vi "Set Relay State.vi"(8 "error in (no error)":errorcluster, 9 "relay action (Close Relay)":T1=enum."Close Relay", 10 "SLSC Switch in":refnum<class "SLSC Switch.lvclass">, 11 "DevicePropertyRelay in":refnum<class "DevicePropertyRelay.lvclass">) -> (0 "error out":errorcluster, 2 "SLSC Switch out":refnum<class "SLSC Switch.lvclass">, 3 "DevicePropertyRelay out":refnum<class "DevicePropertyRelay.lvclass">)   [LabVIEW 2015, in "DevicePropertyRelay.lvclass"]
uses:
  DevicePropertyRelay.lvclass
  slscsl/RelayAction.ctl
  SLSC Switch/SLSC Switch.lvclass
  SLSC Switch/SLSC Switch.lvclass/SLSC Switch.ctl
  DevicePropertyRelay.lvclass/DevicePropertyRelay.ctl
  <vilib>/SLSC/Set Device Property (Bool).vi
  <vilib>/SLSC/Commit Properties for Devices.vi
  <vilib>/SLSC/Execute Device Command.vi
  slscsl/slscsl.lvclass
  <vilib>/SLSC/SLSC.lvlib
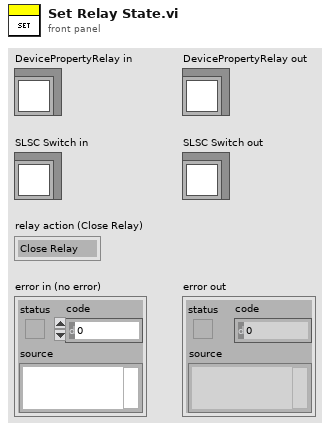
[diagram p1: front panel]
types:
  T1 = typedef "slscsl.lvclass/RelayAction.ctl" = enum16{"Open Relay", "Close Relay"}
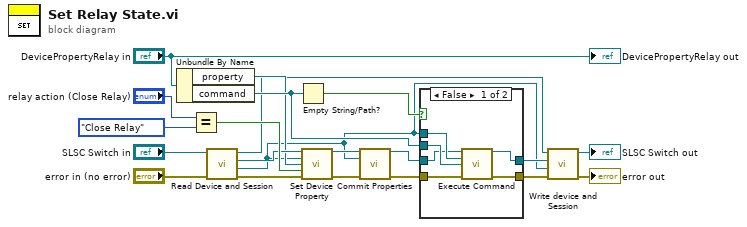
[diagram p0: block diagram]
diagram:
  n1 = Unbundle By Name("DevicePropertyRelay in") -> ("property"=w11:refnum<k21>, "command"=w20:refnum<k21>)
  n2 = Equal?(x="relay action (Close Relay)", y=RelayAction."Close Relay") -> (x = y?=w17:bool)
  n3 = call "Read Device and Session.vi"("error in (no error)"="error in (no error)", "SLSC Switch in"="SLSC Switch in") -> ("error out"=w3:errorcluster, "device"=w5:refnum<k21>, "session"=w12:refnum<k21>, "SLSC Switch out"=w8:refnum<class "SLSC Switch.lvclass">)  [unwired: 6 in]
  n4 = Empty String/Path?(string/path=w20) -> (empty?=w19:bool)
  n5 = call-poly <vilib>:"Set Device Property.vi"("session in"=w12, "devices"=w5, "property"=w11, "property value"=w17, "error in (no error)"=w3) -> ("session out"=w16:refnum<k21>, "error out"=w15:errorcluster)  [unwired: 9 in]
  n6 = call-poly <vilib>:"Commit Properties.vi"("session in"=w16, "devices"=w5, "error in (no error)"=w15) -> ("session out"=w7:refnum<k21>, "error out"=w2:errorcluster)  [unwired: 11 in]
  n7 = case shown="False" w19 {
    tunnel: w20 -> [w27 _]
    tunnel: w5 -> [w26 _]
    tunnel: w7 -> [w25 w29]
    tunnel: [w24 w29] -> w6
    tunnel: w2 -> [w23 w28]
    tunnel: [w22 w28] -> w1
    frame False {
      n8 = call-poly <vilib>:"Execute Command.vi"("session in"=w25, "devices"=w26, "command"=w27, "error in (no error)"=w23) -> ("session out"=w24:refnum<k21>, "error out"=w22:errorcluster)  [unwired: 10 in]
    }
    frame True {
    }
  }
  n9 = call "Write device and Session.vi"("error in (no error)"=w1, "device"=w5, "session"=w6, "SLSC Switch in"=w8) -> ("error out"=→"error out":errorcluster, "SLSC Switch out"=→"SLSC Switch out":refnum<class "SLSC Switch.lvclass">)  [unwired: 6 in]
  "DevicePropertyRelay out" <- "DevicePropertyRelay in"
